vi "test.vi"() -> ()   [LabVIEW 2025, in "Rigol.lvlib"]
uses:
  Rigol.lvlib
panel:
  out "value out":errorcluster
  out "error out":errorcluster
  in  "error in":errorcluster caption="error in (no error)"
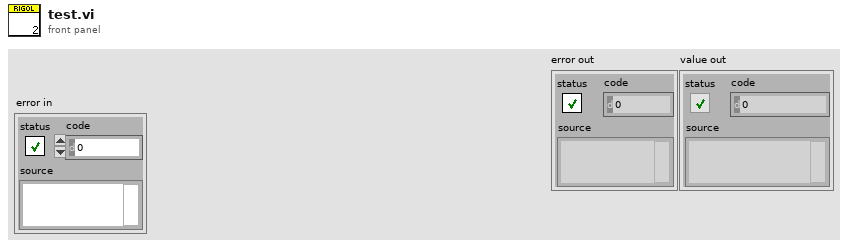
[diagram p1: front panel]
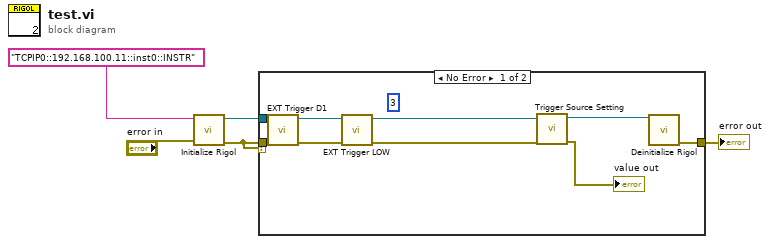
[diagram p0: block diagram]
diagram:
  n1 = call "Initialize Rigol.vi"("error in"="error in", "Adress"="TCPIP0::192.168.100.11::inst0::INSTR") -> ("error out"=w2:errorcluster, "VISA resource name out"=w4:refnum<visa-resource-name>)  [unwired: 6 in]
  n2 = case shown="No Error" w2 {
    tunnel: w4 -> [w14 _]
    tunnel: w2 -> [w13 w15]
    tunnel: [w9 w15] -> w3
    frame No Error {
      (unwired) 3
      n3 = call "EXT Trigger D1.vi"("error in (no error)"=w13, "VISA resource name"=w14) -> ("value out"=w6:errorcluster, "VISA resource name out"=w7:refnum<visa-resource-name>)  [unwired: 8 in]
      n4 = call "EXT Trigger LOW.vi"("error in (no error)"=w6, "VISA resource name"=w7) -> ("value out"=w11:errorcluster, "VISA resource name out"=w12:refnum<visa-resource-name>)  [unwired: 8 in]
      n5 = call "Trigger Source Setting.vi"("error in (no error)"=w11, "VISA resource name"=w12) -> ("value out"=→"value out":errorcluster, "VISA resource name out"=w10:refnum<visa-resource-name>)  [unwired: 8 in]
      n6 = call "Deinitialize Rigol.vi"("VISA resource name"=w10) -> ("error out"=w9:errorcluster)  [unwired: 8 in]
    }
    frame Error {
    }
  }
  "error out" <- w3
